vi "Begin.vi"(8 "error in":errorcluster) -> (0 "error out":errorcluster)   [LabVIEW 2014]
doc: "Called before other user functions, this VI is expected to open initial I/O refnums, load in file data, and do all program initialization. Notice that the <B>error out</B> terminal is simply used for data flow. Wiring it to other structures or subVIs ensures that this VI runs first."
uses:
  <vilib>/Rock Robotics/WPI/SafetyOutput/WPI_SafetyOutputConfigMenu.ctl
  <vilib>/Rock Robotics/WPI/DriverStation/WPI_DriverStationRobotMode2.ctl
  <vilib>/Rock Robotics/WPI/Joystick/WPI_JoystickDeviceEnum.ctl
  <vilib>/Rock Robotics/SystemInterfaces/DIO/FPGA_DIOPWMChannel.ctl
  <vilib>/Rock Robotics/WPI/Solenoid/WPI_SolenoidChannel.ctl
  <vilib>/Rock Robotics/WPI/CAN/TalonSRX/WPI_CANTalonSRX_APIControlMode.ctl
  <vilib>/Rock Robotics/WPI/CAN/TalonSRX/WPI_CANTalonSRX_APIFeedbackSelect.ctl
  <vilib>/Rock Robotics/SystemInterfaces/AI/FPGA_AIChannel.ctl
  <vilib>/Rock Robotics/WPI/CAN/TalonSRX/WPI_CANTalonSRX_BrakeOverride.ctl
  <vilib>/Rock Robotics/SystemInterfaces/AI/FPGA_AIGyroChannel.ctl
  <vilib>/Rock Robotics/SystemInterfaces/DIO/FPGA_DIOChannel.ctl
  <vilib>/Rock Robotics/WPI/Encoder/WPI_EncoderType.ctl
  Robot Global Data.vi
  <vilib>/Rock Robotics/Network Tables/SD Write String Array.vi
  <vilib>/Rock Robotics/WPI/Solenoid/WPI_SolenoidOpenDouble.vi
  <vilib>/Rock Robotics/WPI/RobotDrive/WPI_RobotDriveOpen4MotorWithTalon.vi
  <vilib>/Rock Robotics/WPI/MotorControl/WPI_MotorControlOpenCANTalonSRX.vi
  <vilib>/Rock Robotics/WPI/Counter/WPI_CounterDigitalInputToDigitalSource.vi
  <vilib>/Rock Robotics/WPI/Compressor/WPI_CompressorGetSetRefNum.vi
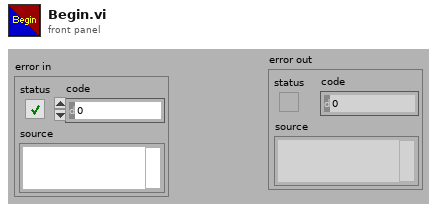
[diagram p1: front panel]
types:
  T1 = typedef "WPI_EncoderType.ctl" = enum16{"1x", "2x", "4x"}
  T2 = typedef "FPGA_DIOChannel.ctl" = enum8{"DIO 0", "DIO 1", "DIO 2", "DIO 3", "DIO 4", "DIO 5", "DIO 6", "DIO 7", "DIO 8", "DIO 9", "DIO MXP 0", "DIO MXP 1", "DIO MXP 2", "DIO MXP 3", "DIO MXP 4", "DIO MXP 5", "DIO MXP 6", "DIO MXP 7", "DIO MXP 8", "DIO MXP 9", "DIO MXP 10", "DIO MXP 11", "DIO MXP 12", "DIO MXP 13", "DIO MXP 14", "DIO MXP 15", "Invalid"}
  T3 = typedef "WPI_SolenoidChannel.ctl" = enum8{"Solenoid 0", "Solenoid 1", "Solenoid 2", "Solenoid 3", "Solenoid 4", "Solenoid 5", "Solenoid 6", "Solenoid 7", "Invalid"}
  T4 = typedef "FPGA_AIGyroChannel.ctl" = enum8{"AI 0", "AI 1", "Invalid"}
  T5 = typedef "WPI_JoystickDeviceEnum.ctl" = enum16{"USB 0", "USB 1", "USB 2", "USB 3", "USB 4", "USB 5"}
  T6 = typedef "WPI_CANTalonSRX_BrakeOverride.ctl" = enum8{"No Override", "Override to Coast", "Override to Brake"}
  T7 = typedef "FPGA_AIChannel.ctl" = enum8{"AI 0", "AI 1", "AI 2", "AI 3", "AI MXP 0", "AI MXP 1", "AI MXP 2", "AI MXP 3", "Invalid"}
  T8 = typedef "WPI_CANTalonSRX_APIFeedbackSelect.ctl" = enum16{"Digital Quadrature Encoder", "Analog Potentiometer", "Analog Encoder"}
  T9 = typedef "WPI_CANTalonSRX_APIControlMode.ctl" = enum8{"Percent VBus", "Speed", "Position", "Slave", "Unchanged / Invalid"}
  T10 = typedef "FPGA_DIOPWMChannel.ctl" = enum8{"PWM 0", "PWM 1", "PWM 2", "PWM 3", "PWM 4", "PWM 5", "PWM 6", "PWM 7", "PWM 8", "PWM 9", "PWM MXP 0", "PWM MXP 1", "PWM MXP 2", "PWM MXP 3", "PWM MXP 4", "PWM MXP 5", "PWM MXP 6", "PWM MXP 7", "PWM MXP 8", "PWM MXP 9", "Invalid"}
  T11 = typedef "WPI_DriverStationRobotMode2.ctl" = enum16{"Autonomous Disabled", "Autonomous Enabled", "Teleop Disabled", "Teleop Enabled", "Disconnected", "Finish", "Test Disabled", "Test Enabled", "Emergency Stopped"}
  T12 = typedef "WPI_SafetyOutputConfigMenu.ctl" = enum16{"Enable", "Disable"}
  T13 = typedef "WPI_JoystickDevRef.ctl" = cluster{"Device":T5}
  T14 = typedef "WPI_RobotDriveDevRef.ctl" = cluster{"DevStatus":errorcluster, "Motors[]":T15[], "Square Inputs":bool, "Max Output":dbl}
  T15 = typedef "WPI_MotorControlDeviceRef.ctl" = cluster{"DeviceStatus":errorcluster, "Type":T16, "PWM":cluster{"Controller":T17, "PWM Channel":T10, "DeadBand":T18}, "CAN":cluster{"Device Number":u8, "Control Mode":T19, "Semaphore":T20, "Max Vout":dbl, "TalonSRX Control Mode":T9}, "Invert":bool, "TransformRef":T21, "InvTransformRef":T21}
  T16 = typedef "WPI_MotorControlType.ctl" = enum16{"PWM", "CAN", "CANTalonSRX"}
  T17 = typedef "FPGA_TypedefDigitalModule.ctl" = enum16{"Controller 1"}
  T18 = typedef "WPI_PWMDeadband.ctl" = cluster{"Name":string, "maxPositivePwm":i32, "minPositivePwm":i32, "centerPwm":i32, "maxNegativePwm":i32, "minNegativePwm":i32, "angularRange":u16}
  T19 = typedef "WPI_CANJaguar_ControlMode.ctl" = enum8{"Percent VBus", "Current", "Speed", "Position", "Voltage"}
  T20 = typedef "Semaphore RefNum" = refnum<k1>
  T21 = typedef "WPI_PWMTransform_ConPane.ctl" = refnum<vi>
  T22 = typedef "WPI_SolenoidDevRef.ctl" = cluster{"DevStatus":errorcluster, "Pneumatics Control Module":u8, "Forward Solenoid Channel":T3, "Reverse Solenoid Channel":T3}
  T23 = typedef "WPI_DigitalInputDevRef.ctl" = cluster{"DevStatus":errorcluster, "DIO Channel":T2, "Controller":T17}
  T24 = typedef "WPI_CompressorDevRef.ctl" = cluster{"DevStatus":errorcluster, "Pneumatics Control Module":u8}
  T25 = typedef "WPI_GyroDevRef.ctl" = cluster{"DevStatus":errorcluster, "Analog Module":T26, "Analog Channel":T7, "Offset":dbl, "Gain (VoltsPerDegree/Second)":dbl}
  T26 = typedef "FPGA_TypedefAnalogModule.ctl" = enum16{"Controller 1"}
  T27 = typedef "WPI_AnalogChannelDevRef.ctl" = cluster{"DevStatus":errorcluster, "Controller":T26, "Analog Channel":T7}
  T28 = typedef "FPGA_CounterEncoderSourceConvertionLVSourceType.ctl" = cluster{"DevStatus":errorcluster, "AnalogTriggerMode?":bool, "DigitalMode":cluster{"Controller":T17, "DIO Channel":T29}, "AnalogTriggerMode":cluster{"AnalogTriggerIndex":T30, "OutputType":T31}}
  T29 = typedef "FPGA_DIODigitalSourceChannel.ctl" = enum8{"DIO 0", "DIO 1", "DIO 2", "DIO 3", "DIO 4", "DIO 5", "DIO 6", "DIO 7", "DIO 8", "DIO 9", "DIO MXP 0", "DIO MXP 1", "DIO MXP 2", "DIO MXP 3", "DIO MXP 4", "DIO MXP 5", "DIO MXP 6", "DIO MXP 7", "DIO MXP 8", "DIO MXP 9", "DIO MXP 10", "DIO MXP 11", "DIO MXP 12", "DIO MXP 13", "DIO MXP 14", "DIO MXP 15", "Disabled"}
  T30 = typedef "FPGA_AnalogTriggerIndex.ctl" = enum8{"Trig 0", "Trig 1", "Trig 2", "Trig 3", "Trig 4", "Trig 5", "Trig 6", "Trig 7", "Invalid"}
  T31 = typedef "FPGA_AnalogTriggerOutType.ctl" = enum16{"InWindow", "TriggerState", "Rising", "Falling"}
  T32 = typedef "WPI_EncoderDevRef.ctl" = cluster{"DevStatus":errorcluster, "EncoderIndex":T33, "CounterIndex":T34, "DistancePerCount":dbl, "Decoding Type":T1}
  T33 = typedef "FPGA_EncoderIdx.ctl" = enum8{"Enc 0", "Enc 1", "Enc 2", "Enc 3", "Enc 4", "Enc 5", "Enc 6", "Enc 7", "Invalid"}
  T34 = typedef "FPGA_CounterCtrSystemIndex.ctl" = enum8{"Ctr 0", "Ctr 1", "Ctr 2", "Ctr 3", "Ctr 4", "Ctr 5", "Ctr 6", "Ctr 7", "Invalid"}
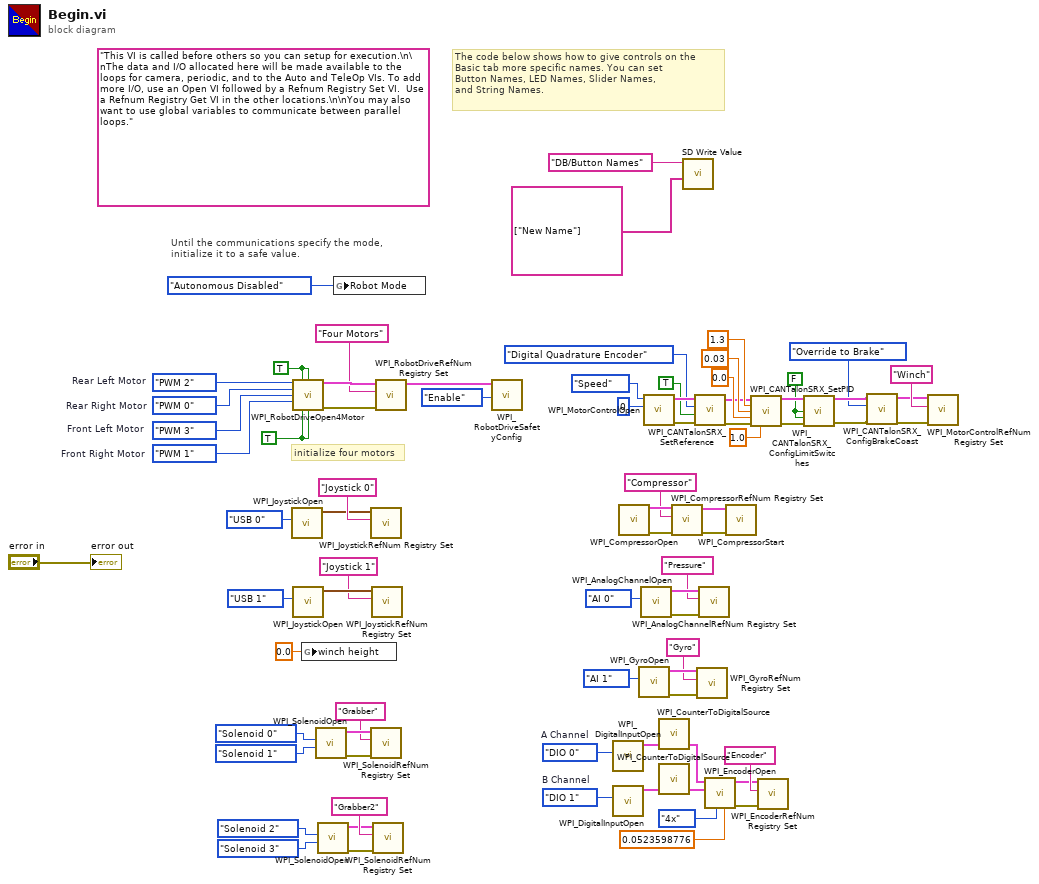
[diagram p0: block diagram]
diagram:
  w13 = FPGA_DIOChannel."DIO 1"  # B Channel
  w12 = FPGA_DIOChannel."DIO 0"  # A Channel
  w2 = FALSE ("Forward Limit Switch Normally Open")
  w49 = TRUE ("Front Left Motor Inverted")
  w50 = TRUE ("Rear Right Motor Inverted")
  w65 = FPGA_DIOPWMChannel."PWM 1"  # Front Right Motor
  w66 = FPGA_DIOPWMChannel."PWM 3"  # Front Left Motor
  w67 = FPGA_DIOPWMChannel."PWM 0"  # Rear Right Motor
  w68 = FPGA_DIOPWMChannel."PWM 2"  # Rear Left Motor
  (unwired) "This VI is called before others so you can setup for execution.\n\nThe data and I/O allocated here will be made available to the loops for camera, periodic, and to the Auto and TeleOp VIs. To add more I/O, use an Open VI followed by a Refnum Registry Set VI.  Use a Refnum Registry Get VI in the other locations.\n\nYou may also want to use global variables to communicate between parallel loops."
  # "The code below shows how to give controls on the\nBasic tab more specific names. You can set\nButton Names, LED Names, Slider Names,\nand String Names."
  # "Until the communications specify the mode,\ninitialize it to a safe value."
  # "initialize four motors"
  n1 = call <vilib>:"WPI_JoystickOpen.vi"("JoystickDevice"=WPI_JoystickDeviceEnum."USB 0") -> ("JoystickDevRef"=w70:T13)  [unwired: 10 in]
  n2 = call-poly <vilib>:"WPI_RobotDriveOpen4Motor.vi"("Rear Left Motor"=w68, "Rear Left Motor Inverted"=w50, "Rear Right Motor Inverted"=w50, "Rear Right Motor"=w67, "Front Left Motor"=w66, "Front Right Motor"=w65, "Front Left Motor Inverted"=w49, "Front Right Motor Inverted"=w49) -> ("RobotDriveDevRef"=w77:T14, "error out"=w75:errorcluster)  [unwired: 6 in]
  n3 = call <vilib>:"WPI_JoystickOpen.vi"("JoystickDevice"=WPI_JoystickDeviceEnum."USB 1") -> ("JoystickDevRef"=w24:T13)  [unwired: 10 in]
  n4 = global write "Robot Global Data.vi" "winch height"(0.0 ("winch height")) -> ()
  n5 = call-poly <vilib>:"WPI_SolenoidOpen.vi"("Reverse Solenoid Channel"=WPI_SolenoidChannel."Solenoid 1", "Forward Solenoid Channel"=WPI_SolenoidChannel."Solenoid 0") -> ("error out"=w53:errorcluster, "SolenoidDevRef"=w52:T22)  [unwired: 8 in]
  n6 = call-poly <vilib>:"WPI_SolenoidOpen.vi"("Reverse Solenoid Channel"=WPI_SolenoidChannel."Solenoid 3", "Forward Solenoid Channel"=WPI_SolenoidChannel."Solenoid 2") -> ("error out"=w16:errorcluster, "SolenoidDevRef"=w17:T22)  [unwired: 8 in]
  n7 = global write "Robot Global Data.vi" "Robot Mode"(WPI_DriverStationRobotMode2."Autonomous Disabled" ("Robot Mode")) -> ()
  n8 = call <vilib>:"WPI_JoystickRefNum Registry Set.vi"("refnum name"="Joystick 0", "JoystickDevRef"=w70) -> ()  [unwired: 8 in, 2 out]
  n9 = call <vilib>:"WPI_SolenoidRefNum Registry Set.vi"("error in (no error)"=w53, "refnum name"="Grabber", "SolenoidDevRef"=w52) -> ()  [unwired: 7 in, 2 out]
  n10 = call <vilib>:"WPI_JoystickRefNum Registry Set.vi"("refnum name"="Joystick 1", "JoystickDevRef"=w24) -> ()  [unwired: 8 in, 2 out]
  n11 = call <vilib>:"WPI_SolenoidRefNum Registry Set.vi"("error in (no error)"=w16, "refnum name"="Grabber2", "SolenoidDevRef"=w17) -> ()  [unwired: 7 in, 2 out]
  n12 = call <vilib>:"WPI_RobotDriveRefNum Registry Set.vi"("error in (no error)"=w75, "refnum name"="Four Motors", "RobotDriveDevRef"=w77) -> ("RobotDriveDevRef"=w74:T14)  [unwired: 8 out]
  n13 = call <vilib>:"WPI_RobotDriveSafetyConfig.vi"("mode"=WPI_SafetyOutputConfigMenu."Enable", "RobotDriveDevRef"=w74) -> ()  [unwired: 8 in, 2 out]
  n14 = call <vilib>:"WPI_DigitalInputOpen.vi"("DIO Channel"=w12) -> ("DigitalInputDevRef"=w9:T23)  [unwired: 2 in, 8 out]
  n15 = call <vilib>:"WPI_DigitalInputOpen.vi"("DIO Channel"=w13) -> ("DigitalInputDevRef"=w10:T23)  [unwired: 2 in, 8 out]
  n16 = call <vilib>:"WPI_CompressorOpen.vi"() -> ("CompressorDevRef"=w59:T24, "error out"=w60:errorcluster)  [unwired: 14 in]
  n17 = call <vilib>:"WPI_GyroOpen.vi"("Analog Channel"=FPGA_AIGyroChannel."AI 1") -> ("error out"=w22:errorcluster, "GyroDevRef"=w21:T25)  [unwired: 8 in, 1 out]
  n18 = call <vilib>:"WPI_AnalogChannelOpen.vi"("Analog Channel"=FPGA_AIChannel."AI 0") -> ("error out"=w37:errorcluster, "AIDeviceRef"=w36:T27)  [unwired: 9 in]
  n19 = call-poly <vilib>:"WPI_MotorControlOpen.vi"("Device Number"=u8 0, "Control Mode"=WPI_CANTalonSRX_APIControlMode."Speed") -> ("error out"=w43:errorcluster, "MotorControlDeviceRef"=w42:T15)  [unwired: 8 in]
  n20 = call-poly <vilib>:"WPI_CounterToDigitalSource.vi"("DigitalInputDevRef"=w9) -> ("Digital Source"=w8:T28)  [unwired: 6 out]
  n21 = call-poly <vilib>:"WPI_CounterToDigitalSource.vi"("DigitalInputDevRef"=w10) -> ("Digital Source"=w11:T28)  [unwired: 6 out]
  n22 = call <vilib>:"WPI_CompressorRefNum Registry Set.vi"("error in (no error)"=w60, "refnum name"="Compressor", "CompressorDevRef"=w59) -> ("error out"=w58:errorcluster, "CompressorDevRef"=w57:T24)  [unwired: 7 in]
  n23 = call-poly <vilib>:"SD Write Value.vi"("String Array"=string[] ["New Name"], "Name"="DB/Button Names") -> ()  [unwired: 8 in, 2 out]
  n24 = call <vilib>:"WPI_CANTalonSRX_SetReference.vi"("error in (no error)"=w43, "Reverse Feedback Sensor"=TRUE, "Feedback Reference"=WPI_CANTalonSRX_APIFeedbackSelect."Digital Quadrature Encoder", "CAN Talon SRX Ref"=w42) -> ("error out"=w39:errorcluster, "CAN Talon SRX Ref Out"=w40:T15)  [unwired: 6 in]
  n25 = call <vilib>:"WPI_GyroRefNum Registry Set.vi"("error in (no error)"=w22, "refnum name"="Gyro", "GyroDevRef"=w21) -> ()  [unwired: 7 in, 2 out]
  n26 = call <vilib>:"WPI_AnalogChannelRefNum Registry Set.vi"("error in (no error)"=w37, "refnum name"="Pressure", "AIDeviceRef"=w36) -> ()  [unwired: 7 in, 2 out]
  n27 = call <vilib>:"WPI_EncoderOpen.vi"("DistancePerCount"=0.0523598776, "Decoding Type"=WPI_EncoderType."4x", "BSource"=w11, "ASource"=w8) -> ("error out"=w4:errorcluster, "EncoderDevRef"=w3:T32)  [unwired: 4 in, 2 out]
  n28 = call <vilib>:"WPI_CompressorStart.vi"("error in (no error)"=w58, "CompressorDevRef"=w57) -> ()  [unwired: 8 in, 2 out]
  n29 = call <vilib>:"WPI_CANTalonSRX_SetPID.vi"("CAN Talon SRX Ref"=w40, "P"=1.3, "I"=0.03, "D"=0.0, "error in (no error)"=w39, "F"=1.0) -> ("CAN Talon SRX Ref Out"=w32:T15, "error out"=w31:errorcluster)  [unwired: 8 in]
  n30 = call <vilib>:"WPI_EncoderRefNum Registry Set.vi"("error in (no error)"=w4, "refnum name"="Encoder", "EncoderDevRef"=w3) -> ()  [unwired: 7 in, 2 out]
  n31 = call <vilib>:"WPI_CANTalonSRX_ConfigLimitSwitches.vi"("CAN Talon SRX Ref"=w32, "Forward Limit Switch Normally Open"=w2, "Reverse Limit Switch Normally Open"=w2, "error in (no error)"=w31) -> ("CAN Talon SRX Ref Out"=w30:T15, "error out"=w29:errorcluster)  [unwired: 10 in]
  n32 = call <vilib>:"WPI_CANTalonSRX_ConfigBrakeCoast.vi"("error in (no error)"=w29, "Brake / Coast Mode"=WPI_CANTalonSRX_BrakeOverride."Override to Brake", "CAN Talon SRX Ref"=w30) -> ("error out"=w27:errorcluster, "CAN Talon SRX Ref Out"=w28:T15)  [unwired: 7 in]
  n33 = call <vilib>:"WPI_MotorControlRefNum Registry Set.vi"("error in (no error)"=w27, "refnum name"="Winch", "MotorControlDevRef"=w28) -> ()  [unwired: 7 in, 2 out]
  "error out" <- "error in"
